vi "Calculate Ramp Budget.vi"(9 "Rate (T/min)":dbl, 10 "End Field (T)":dbl, 11 "Start Field (T)":dbl) -> (3 "Budget (ms)":u32)   [LabVIEW 2019, in "Instrument.Oxford1820.lvclass"]
uses:
  Instrument.Oxford1820.lvclass
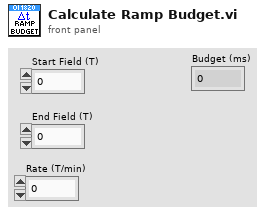
[diagram p1: front panel]
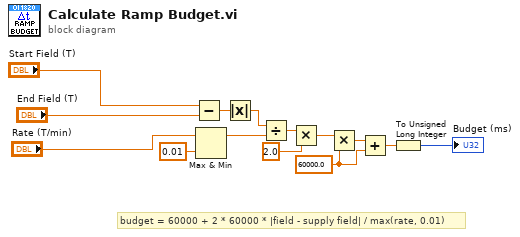
[diagram p0: block diagram]
diagram:
  w13 = 60000.0
  # "budget = 60000 + 2 * 60000 * |field - supply field| / max(rate, 0.01)"
  n1 = Subtract(x="Start Field (T)", y="End Field (T)") -> (x-y=w1:dbl)
  n2 = Max & Min(x="Rate (T/min)", y=0.01) -> (max(x,y)=w4:dbl)  [unwired: 1 out]
  n3 = Absolute Value(x=w1) -> (abs(x)=w2:dbl)
  n4 = Divide(x=w2, y=w4) -> (x/y=w5:dbl)
  n5 = Multiply(x=w5, y=2.0) -> (x*y=w7:dbl)
  n6 = Multiply(x=w7, y=w13) -> (x*y=w8:dbl)
  n7 = Add(x=w8, y=w13) -> (x+y=w9:dbl)
  n8 = To Unsigned Long Integer(number=w9) -> (unsigned 32bit integer=→"Budget (ms)":u32)
